vi "Aiming and Range.vi"() -> ()   [LabVIEW 2019]
panel:
  in  "Right Command":dbl
  in  "Left Command":dbl
  out "Distance Adjust":dbl
  out "Steering Adjust":dbl
  out "Distance Error":dbl
  out "Heading Error":dbl
  in  "ty":dbl
  in  "tx":dbl
  in  "Min Aim Command":dbl=0.05
  in  "KpDistance":dbl=-0.1
  in  "KpAim":dbl=-0.1
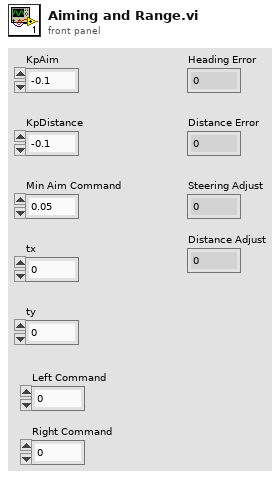
[diagram p1: front panel]
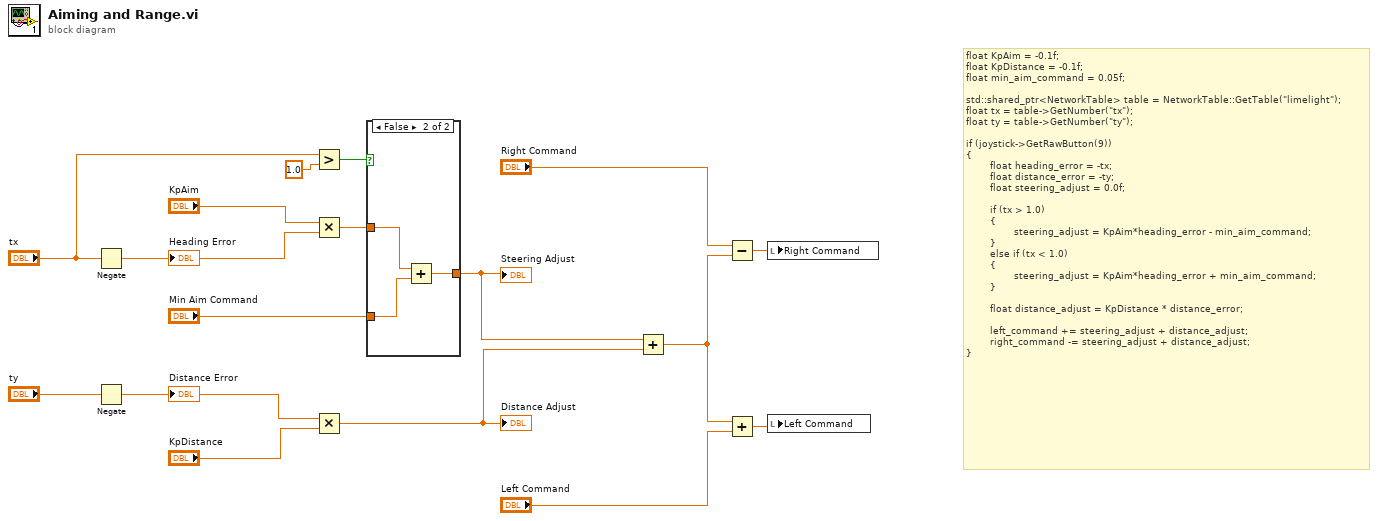
[diagram p0: block diagram]
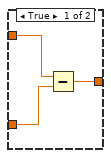
[diagram p2: hidden frame]
diagram:
  # "float KpAim = -0.1f;\nfloat KpDistance = -0.1f;\nfloat min_aim_command = 0.05f;\n\nstd::shared_ptr<NetworkTable> table = NetworkTable::GetTable(\"limelight\");\nfloat tx = table->GetNumber(\"tx\");\nfloat ty = table->GetNumber(\"ty\");\n\nif (joystick->GetRawButton(9))\n{\n        float heading_error = -tx;\n        float distance_error = -ty;\n        float steering_adjust = 0.0f;\n\n        if (tx > 1.0)\n        {\n                steering_adjust = KpAim*heading_error - min_aim_command;\n        }\n        else if (tx < 1.0)\n        {\n                steering_adjust = KpAim*heading_error + min_aim_command;\n        }\n\n        float distance_adjust = KpDistance * distance_error;\n\n        left_command += steering_adjust + distance_adjust;\n        right_command -= steering_adjust + distance_adjust;\n}"
  n1 = Negate(x="tx") -> (-x=w12:dbl)
  "Heading Error" <- w12
  n2 = Negate(x="ty") -> (-x=w8:dbl)
  "Distance Error" <- w8
  n3 = Greater?(x="tx", y=1.0) -> (0:w14:bool)
  n4 = Multiply(x="KpAim", y=w12) -> (x*y=w11:dbl)
  n5 = Multiply(x=w8, y="KpDistance") -> (x*y=w6:dbl)
  "Distance Adjust" <- w6
  n6 = case shown="False" w14 {
    tunnel: w11 -> [w20 w23]
    tunnel: "Min Aim Command" -> [w19 w22]
    tunnel: [w18 w21] -> w7
    frame True {
      n7 = Subtract(x=w20, y=w19) -> (x-y=w18:dbl)
    }
    frame False {
      n8 = Add(x=w23, y=w22) -> (x+y=w21:dbl)
    }
  }
  "Steering Adjust" <- w7
  n9 = Add(x=w7, y=w6) -> (x+y=w2:dbl)
  n10 = Subtract(x="Right Command", y=w2) -> (x-y=w1:dbl)
  n11 = Add(x=w2, y="Left Command") -> (x+y=w5:dbl)
  n12 = local write "Right Command"(w1) -> ()
  n13 = local write "Left Command"(w5) -> ()
